vi "Close_camera.vi"(8 "error in":errorcluster, 11 "camera handle in":u64) -> (0 "error out":errorcluster)   [LabVIEW 2019, in "PICam.lvlib"]
doc: "Picam_CloseCamera() releases all resources that have been associated with a specified\ncamera.\n\nNote: Prior to program termination (and before calling the \"Uninit_library.vi\"), all open cameras must be closed by calling Picam_CloseCamera()."
uses:
  PICam.lvlib
  Picam64.dll   
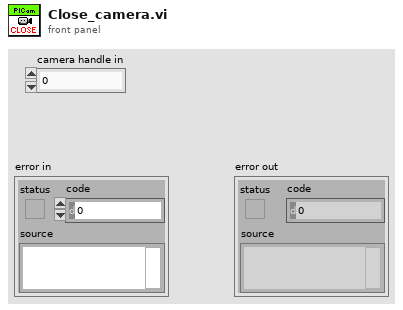
[diagram p1: front panel]
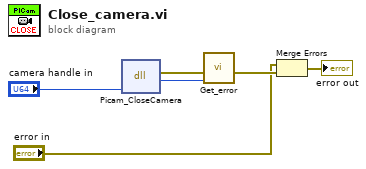
[diagram p0: block diagram]
diagram:
  n1 = dll-call lib="Picam32.dll" fn="Picam_CloseCamera"("camera"="camera handle in") -> (error out=w5:errorcluster, "return type"=w4:i32)  [unwired: 4 in, 1 out]
  n2 = call "Get_error.vi"("PICam_Error"=w4, "error in (no error)"=w5) -> ("error out"=w6:errorcluster)  [unwired: 9 in]
  n3 = Merge Errors("error in", w6) -> (→"error out":errorcluster)
